vi "Read Client Count.vi"(11 "Client in":refnum<class "Client.lvclass">) -> (2 "Client Count":i32)   [LabVIEW 2016, in "Client.lvlib" / "Client.lvclass"]
uses:
  Client.lvclass
  Client.lvclass/Client.ctl
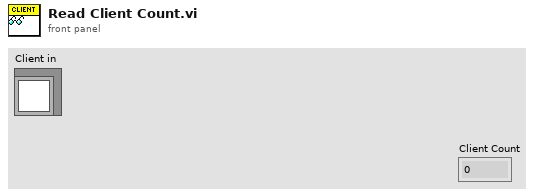
[diagram p1: front panel]
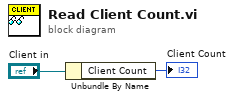
[diagram p0: block diagram]
diagram:
  n1 = Unbundle By Name("Client in") -> ("Client Count"=→"Client Count":i32)
